vi "PopulateDBAutoSelectors.vi"(3 "Reload Routines":bool, 4 "Auto Routines Storage Directory":path=path "/home/lvuser/AutoRoutines", 5 "MotionPlanningNotifiers":T1, 6 "DefaultStartingPosition":T12) -> (0 "AllRoutines":T2 {"Routines"."ArmPath"."ExtendTrajectory"."Time (ms)" items=["TrajectoryDuration_0ms"=0, "TrajectoryDuration_5ms"=5, "TrajectoryDuration_10ms"=10, "TrajectoryDuration_20ms"=20, "TrajectoryDuration_30ms"=30, "TrajectoryDuration_40ms"=40, "TrajectoryDuration_50ms"=50, "TrajectoryDuration_100ms"=100]; "Routines"."ArmPath"."RotateTrajectory"."Time (ms)" items=["TrajectoryDuration_0ms"=0, "TrajectoryDuration_5ms"=5, "TrajectoryDuration_10ms"=10, "TrajectoryDuration_20ms"=20, "TrajectoryDuration_30ms"=30, "TrajectoryDuration_40ms"=40, "TrajectoryDuration_50ms"=50, "TrajectoryDuration_100ms"=100]}, 1 "AvailableRoutines":T2 {"Routines"."ArmPath"."ExtendTrajectory"."Time (ms)" items=["TrajectoryDuration_0ms"=0, "TrajectoryDuration_5ms"=5, "TrajectoryDuration_10ms"=10, "TrajectoryDuration_20ms"=20, "TrajectoryDuration_30ms"=30, "TrajectoryDuration_40ms"=40, "TrajectoryDuration_50ms"=50, "TrajectoryDuration_100ms"=100]; "Routines"."ArmPath"."RotateTrajectory"."Time (ms)" items=["TrajectoryDuration_0ms"=0, "TrajectoryDuration_5ms"=5, "TrajectoryDuration_10ms"=10, "TrajectoryDuration_20ms"=20, "TrajectoryDuration_30ms"=30, "TrajectoryDuration_40ms"=40, "TrajectoryDuration_50ms"=50, "TrajectoryDuration_100ms"=100]}, 2 "StartingPosition":T12)   [LabVIEW 2017]
uses:
  Autonomous/TypeDef/AutoStartingPositions.ctl
  Autonomous/TypeDef/AutoRoutineSet.ctl
  Autonomous/TypeDef/AutoPreProcessedStep.ctl
  Autonomous/PathPlannerSupport/TypeDefs/DrivePlanResponse.ctl
  Pathfinder/Pathfinder-LabVIEW/Pathfinder-Lib/VIs/Segment.ctl
  Implements/Arm/TypeDefs/ArmPlanResponse.ctl
  General/MotionProfiling/TypeDefs/TrajectoryPoint.ctl
  <vilib>/Rock Robotics/WPI/ThirdParty/Phoenix-LabVIEW/Motor Controller/Controls/CTRE_Phoenix_MotorControl_TrajectoryPointTimeDur.ctl
  Autonomous/TypeDef/AutoWaypointType.ctl
  Implements/Arm/TypeDefs/ArmTargetPosition.ctl
  Implements/TypeDefs/IntakeState.ctl
  TypeDefs/RobotComponents/MotionPlanningNotifiers.ctl
  Autonomous/PathPlannerSupport/TypeDefs/DrivePlanRequest.ctl
  Pathfinder/Pathfinder-LabVIEW/Pathfinder-Lib/VIs/Waypoint.ctl
  Implements/Arm/TypeDefs/ArmPlanRequest.ctl
  ArgosLib/Signal Processing/TypeDefs/EdgeDetector_Type.ctl
  ab172a07-06bd-4a7d-981c-a8533a1e6be2.vi
  <vilib>/Rock Robotics/Network Tables/NT Read Boolean.vi
  <vilib>/Rock Robotics/Network Tables/NT Write String Array.vi
  <vilib>/Rock Robotics/Network Tables/NT Read Number.vi
  ArgosLib/ArgosLib.lvlib
  <vilib>/Utility/Data Type/NI_Data Type.lvlib
  Pathfinder/Pathfinder-LabVIEW/Pathfinder-Lib/Pathfinder.lvlib
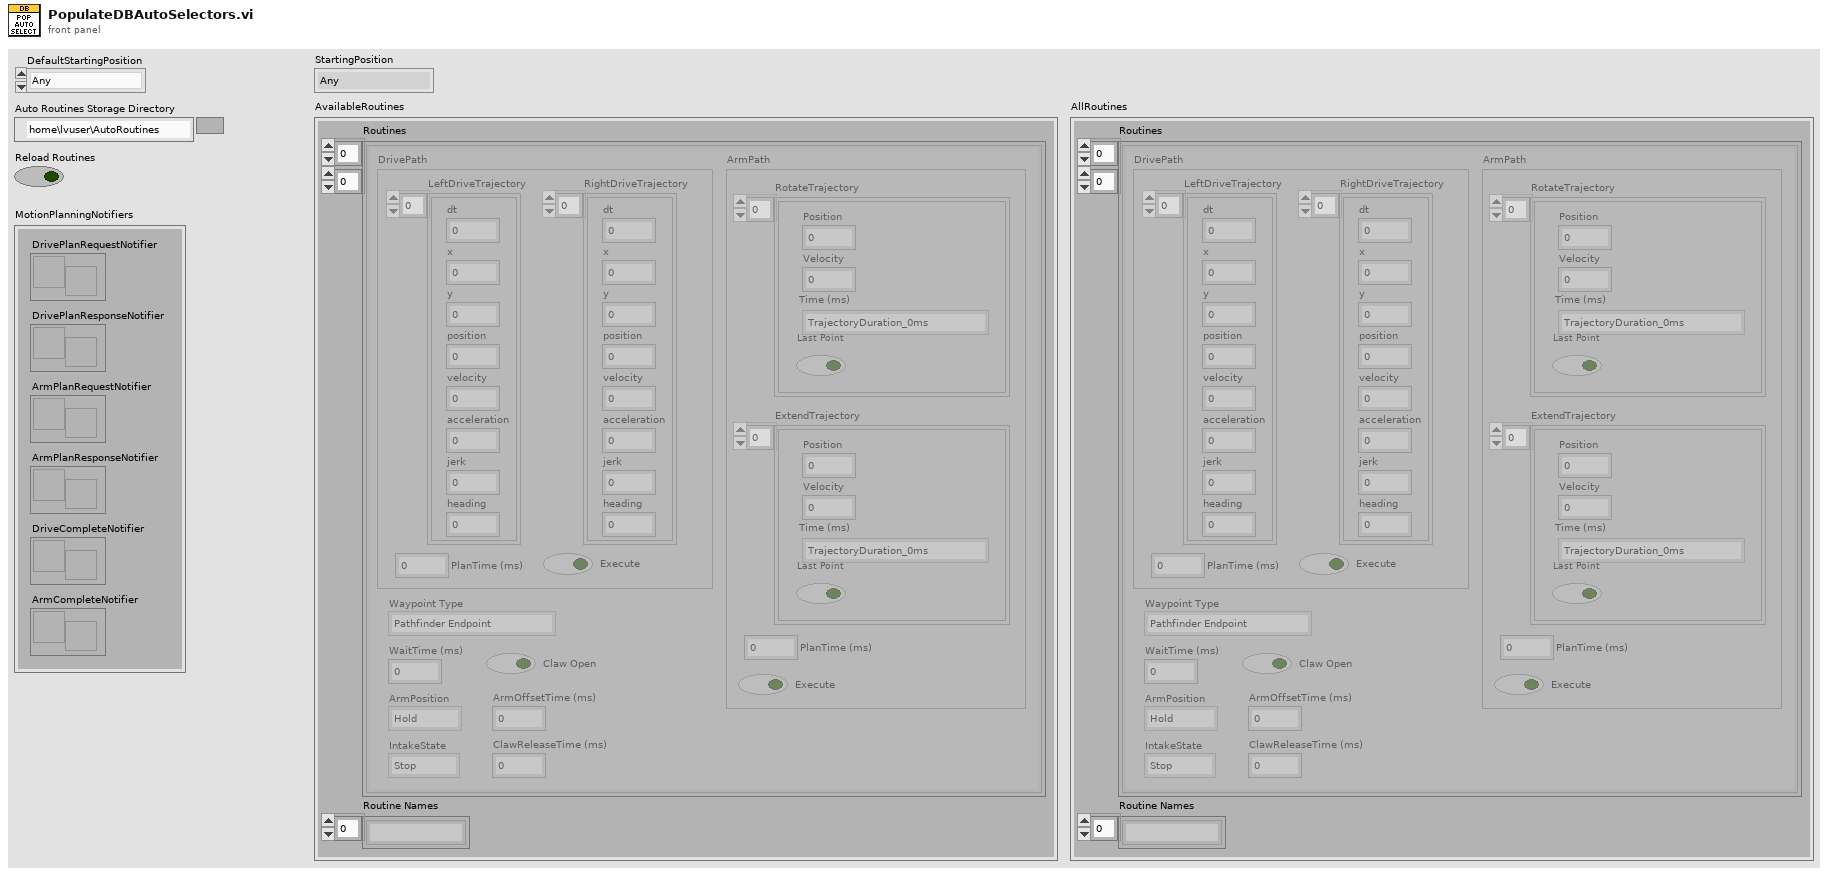
[diagram p1: front panel]
types:
  T1 = typedef "MotionPlanningNotifiers.ctl" = cluster{"DrivePlanRequestNotifier":refnum<notifier>, "DrivePlanResponseNotifier":refnum<notifier>, "ArmPlanRequestNotifier":refnum<notifier>, "ArmPlanResponseNotifier":refnum<notifier>, "DriveCompleteNotifier":refnum<notifier>, "ArmCompleteNotifier":refnum<notifier>}
  T2 = typedef "AutoRoutineSet.ctl" = cluster{"Routine Names":string[], "Routines":T3[][]}
  T3 = typedef "AutoPreProcessedStep.ctl" = cluster{"DrivePath":T4, "ArmPath":T6, "Waypoint Type":T9, "WaitTime (ms)":u16, "ArmPosition":T10, "IntakeState":T11, "Claw Open":bool, "ArmOffsetTime (ms)":u16, "ClawReleaseTime (ms)":i32}
  T4 = typedef "DrivePlanResponse.ctl" = cluster{"LeftDriveTrajectory":T5[], "RightDriveTrajectory":T5[], "PlanTime (ms)":u32, "Execute":bool}
  T5 = typedef "Pathfinder.lvlib/Segment.ctl" = cluster{"dt":dbl, "x":dbl, "y":dbl, "position":dbl, "velocity":dbl, "acceleration":dbl, "jerk":dbl, "heading":dbl}
  T6 = typedef "ArmPlanResponse.ctl" = cluster{"RotateTrajectory":T7[], "ExtendTrajectory":T7[], "PlanTime (ms)":u32, "Execute":bool}
  T7 = typedef "TrajectoryPoint.ctl" = cluster{"Position ":dbl, "Velocity ":dbl, "Time (ms)":T8, "Last Point":bool}
  T8 = typedef "CTRE_Phoenix_MotorControl_TrajectoryPointTimeDur.ctl" = i32
  T9 = typedef "AutoWaypointType.ctl" = enum16{"Pathfinder Endpoint", "Pathfinder Waypoint", "Zero-Radius Turn Endpoint", "Stationary", "Vision Assist Endpoint", "Stop"}
  T10 = typedef "ArmTargetPosition.ctl" = enum16{"Hold", "Switch", "Scale Low", "Scale High", "Climb", "Back Place"}
  T11 = typedef "IntakeState.ctl" = enum16{"Stop", "Forward", "Reverse", "Forward Open"}
  T12 = typedef "AutoStartingPositions.ctl" = enum16{"Any", "Left", "Center", "Right"}
  T13 = typedef "ArgosLib.lvlib/EdgeDetector_Type.ctl" = enum16{"RisingEdge", "FallingEdge", "Both"}
  T14 = typedef "AutoRoutines.ctl" = cluster{"Any Position":T2, "Left Position":T2, "Center Position":T2, "Right Position":T2}
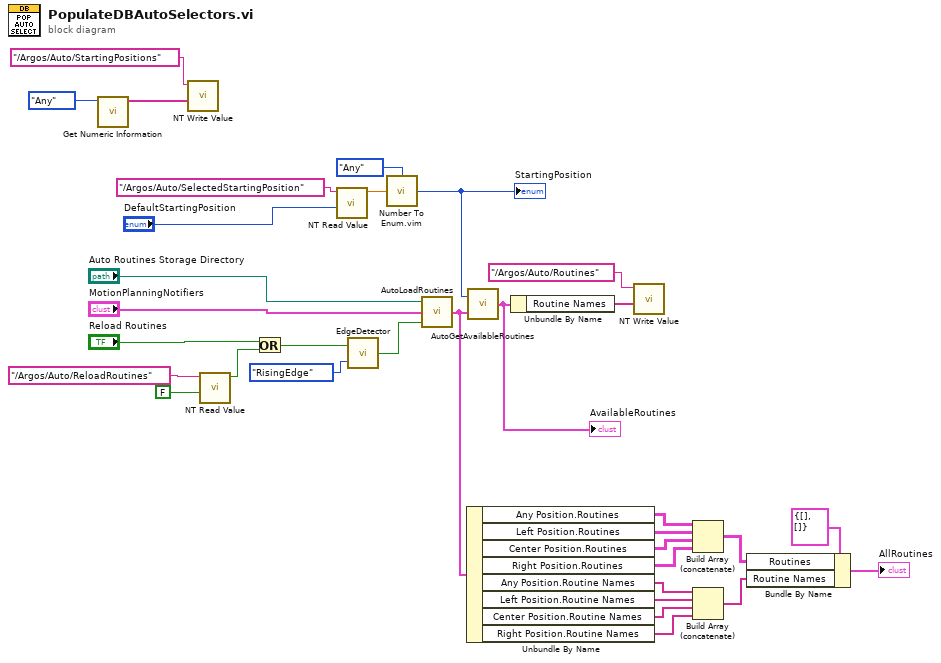
[diagram p0: block diagram]
diagram:
  n1 = call <vilib>:"Get Numeric Information.vi"("Variant"=AutoStartingPositions."Any" ("AutoStartingPosition")) -> ("Enum Names"=w24:string[])  [unwired: 7 in, 3 out]
  n2 = call-poly <vilib>:"NT Write Value.vi"("String Array"=w24, "Name"="/Argos/Auto/StartingPositions") -> ()  [unwired: 9 in, 1 out]
  n3 = call-poly <vilib>:"NT Read Value.vi"("Default Value"=FALSE, "Name"="/Argos/Auto/ReloadRoutines") -> ("Boolean"=w28:bool)  [unwired: 8 in, 1 out]
  n4 = Or(x="Reload Routines", y=w28) -> (x .or. y?=w29:bool)
  n5 = call-poly <vilib>:"NT Read Value.vi"("Default Value"="DefaultStartingPosition", "Name"="/Argos/Auto/SelectedStartingPosition") -> ("Numeric"=w21:dbl)  [unwired: 8 in, 1 out]
  n6 = call "EdgeDetector.vi"("DetectorType"=EdgeDetector_Type."RisingEdge", "Input"=w29) -> ("Edge"=w30:bool)
  n7 = call "Number To Enum.vim"("number"=w21, "enum type"=AutoStartingPositions."Any" ("AutoStartingPosition")) -> ("number as enum"=w20:T12)
  "StartingPosition" <- w20
  n8 = call "AutoLoadRoutines.vi"("Reload Routines"=w30, "MotionPlanningNotifiers"="MotionPlanningNotifiers", "Auto Routines Storage Directory"="Auto Routines Storage Directory") -> ("Auto Routines"=w14:T14)
  n9 = Unbundle By Name(w14) -> ("Any Position.Routines"=w13:T3[][], "Left Position.Routines"=w12:T3[][], "Center Position.Routines"=w11:T3[][], "Right Position.Routines"=w10:T3[][], "Any Position.Routine Names"=w9:string[], "Left Position.Routine Names"=w8:string[], "Center Position.Routine Names"=w7:string[], "Right Position.Routine Names"=w6:string[])
  n10 = call "AutoGetAvailableRoutines.vi"("AllAutoRoutines"=w14, "AutoStartingPosition"=w20) -> ("AvailableRoutines"=w18:T2)
  "AvailableRoutines" <- w18
  n11 = Unbundle By Name(w18) -> ("Routine Names"=w17:string[])
  n12 = call-poly <vilib>:"NT Write Value.vi"("String Array"=w17, "Name"="/Argos/Auto/Routines") -> ()  [unwired: 9 in, 1 out]
  n13 = Build Array (concatenate)(w13, w12, w11, w10) -> (w4:T3[][])
  n14 = Build Array (concatenate)(w9, w8, w7, w6) -> (w3:string[])
  n15 = Bundle By Name(cluster=T2 {"Routine Names"=[], "Routines"=[]} ("AllRoutines"), "Routines"=w4, "Routine Names"=w3) -> (→"AllRoutines":T2)
